vi "Init Events.vi"(8 "error in (no error)":errorcluster, 11 "Editor in":refnum<class "Editor.lvclass">) -> (0 "error out":errorcluster, 3 "Editor out":refnum<class "Editor.lvclass">)   [LabVIEW 2020, in "VolatusGUIEditor.lvlib" / "Editor.lvclass"]
uses:
  Editor.lvclass
  Editor.lvclass/Editor.ctl
  Control Bind Data.ctl
  VolatusGUIControls/VolatusGUIControls.lvlib
  Events.ctl
  Update Preview Data.ctl
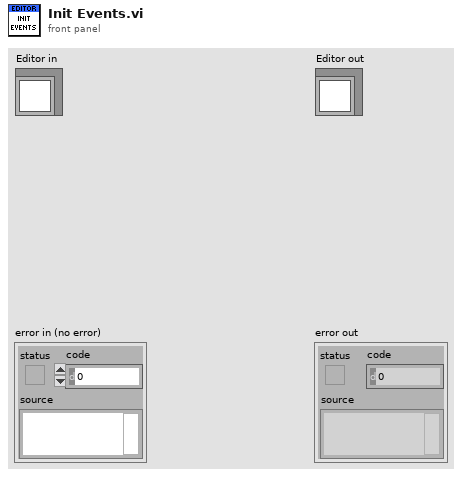
[diagram p1: front panel]
types:
  T1 = typedef "VolatusGUIControls.lvlib/Update Preview Data.ctl" = cluster{"Unused":bool}
  T2 = typedef "VolatusGUIEditor.lvlib/Editor.lvclass/Events.ctl" = cluster{"Update Bind":refnum<user-event>, "Update Preview":refnum<user-event>}
  T3 = typedef "VolatusGUIControls.lvlib/Control Bind Data.ctl" = cluster{"Ctl Refnum":refnum<vi>, "Type Name":string}
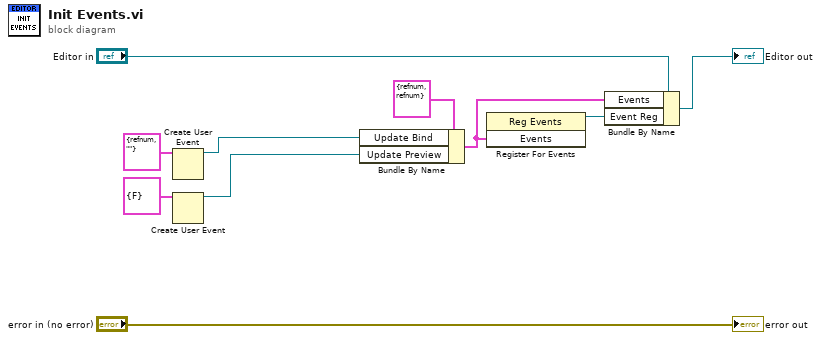
[diagram p0: block diagram]
diagram:
  n1 = Create User Event(user event datatype=T3 {"Ctl Refnum"=refnum, "Type Name"=""} ("Control Bind Data")) -> (user event=w6:refnum<user-event>)  [unwired: 1 in, 1 out]
  n2 = Create User Event(user event datatype=T1 {"Unused"=FALSE} ("Update Preview Data")) -> (user event=w1:refnum<user-event>)  [unwired: 1 in, 1 out]
  n3 = Bundle By Name(cluster=T2 {"Update Bind"=refnum, "Update Preview"=refnum} ("Events"), "Update Bind"=w6, "Update Preview"=w1) -> (w3:T2)
  n4 = register-events(w3) -> (reference out=w4:refnum<event-registration>)  [unwired: 2 in, 1 out]
  n5 = Bundle By Name(cluster="Editor in", "Events"=w3, "Event Reg"=w4) -> (→"Editor out":refnum<class "Editor.lvclass">)
  "error out" <- "error in (no error)"
